vi "Laurel StandAlone TCP.vi"() -> ()   [LabVIEW 2020]
uses:
  Type Definitions/Laurel Serial Commands.ctl
  Type Definitions/Laurel Display Type.ctl
  Type Definitions/Laurel Connection Type.ctl
panel:
  out "appended array":errorcluster[](array[cluster])
  in  "Display Type":T1
  out "Loop Counter":i32
  in  "stop":bool
  out "Single Item":dbl
  out "Gallons (Item 2)":dbl
  out "Flow Rate (Item 1)":dbl format="%.2f"
  in  "All Items Byte Count (Flow Rate)":i32=17
  in  "byte count (Individual)":i32=9
  in  "Laurel Serial Commands":T2
  out "read buffer":string
  out "Error Out 2":errorcluster
  in  "Error In 2":errorcluster
  in  "Hot Laurel Only":string="10.2.0.23"
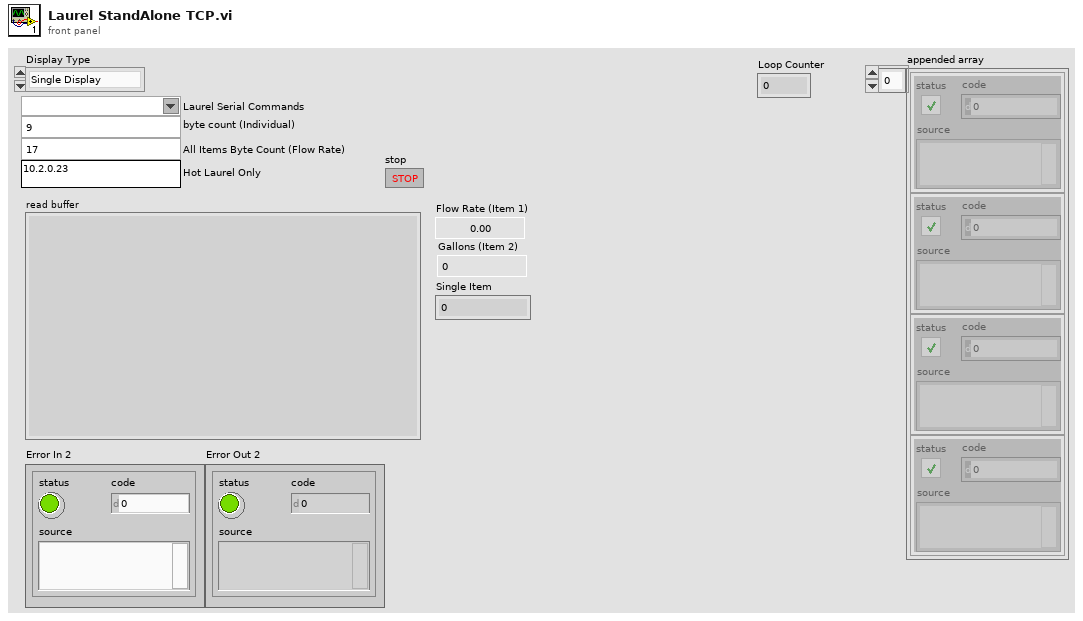
[diagram p1: front panel]
types:
  T1 = typedef "Laurel Display Type.ctl" = enum16{"Single Display", "Dual Display"}
  T2 = typedef "Laurel Serial Commands.ctl" = string
  T3 = typedef "Laurel Connection Type.ctl" = enum16{"Serial", "TCP"}
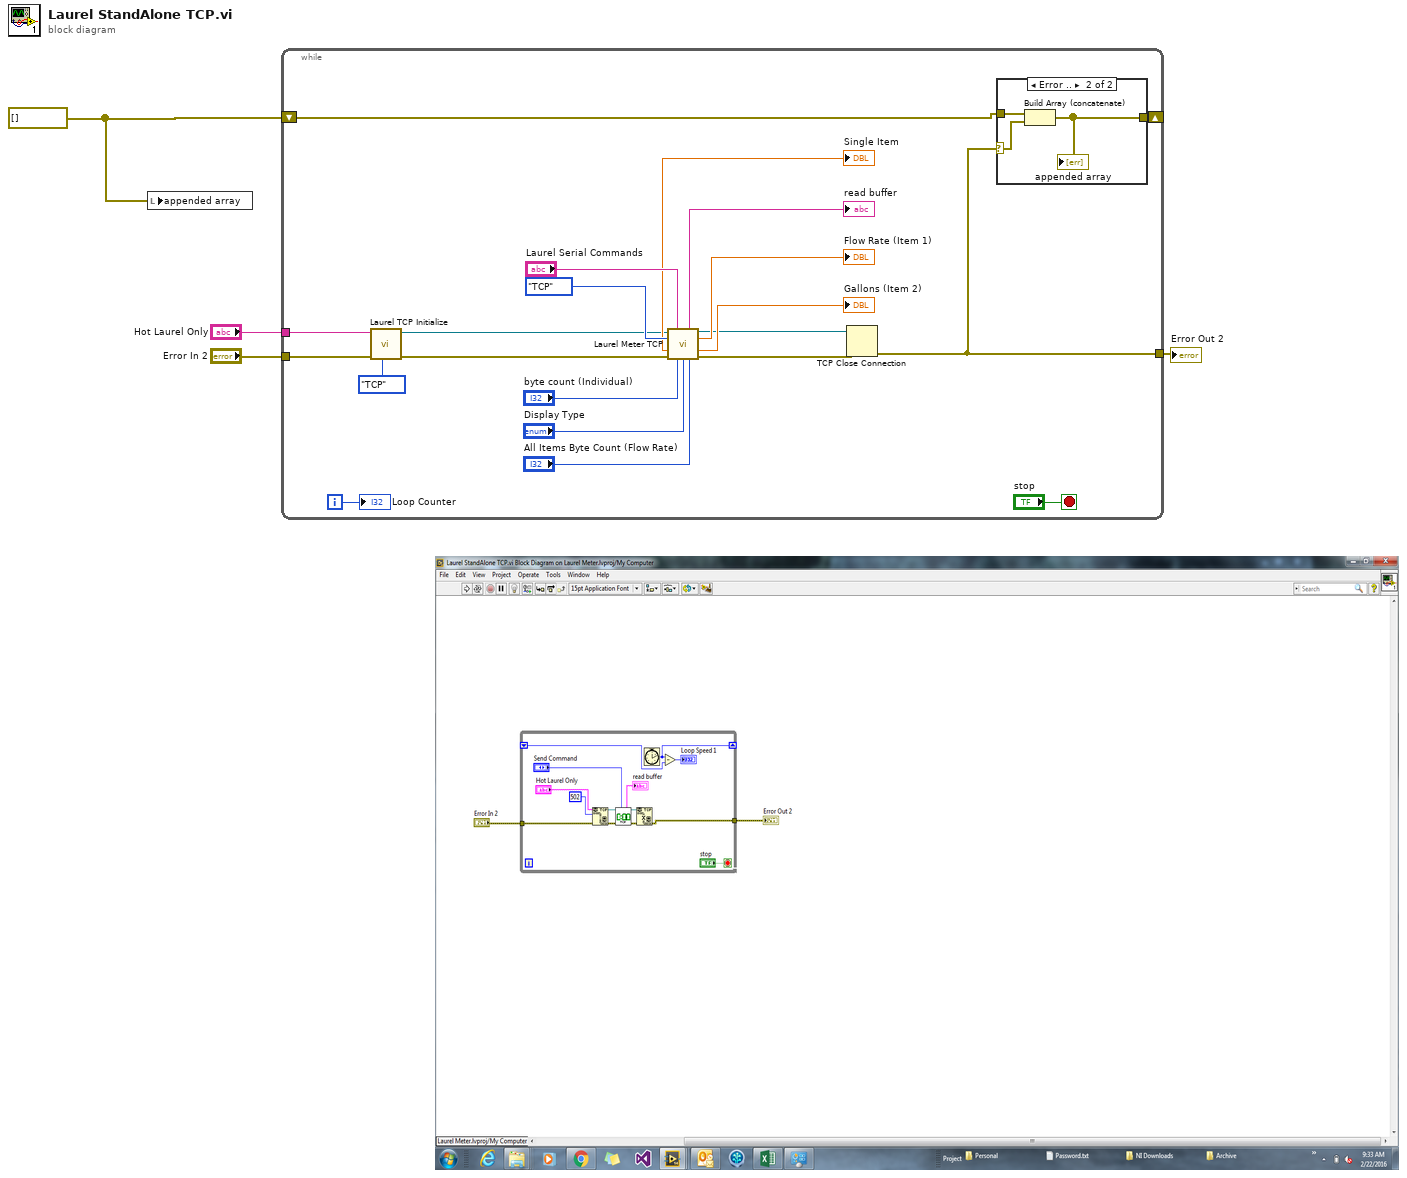
[diagram p0: block diagram]
diagram:
  w1 = errorcluster[] []
  n1 = local write "appended array"(w1) -> ()
  n2 = while {
    tunnel: "Error In 2" -> [w8]
    tunnel: "Hot Laurel Only" -> [w9]
    tunnel: [w11] -> w2
    shift-right: [w10] -> _
    shift-left: w1 -> [w12]
    i -> [w16]
    stop <- "stop" stop-if-true
    n3 = call "Laurel TCP Initialize.vi"("Connection Type"=Laurel_Connection_Type."TCP", "Error In"=w8, "Laurel IP Address"=w9) -> ("Error Out"=w6:errorcluster, "Laurel Ref"=w7:refnum<k5>)  [unwired: 6 in, 1 out]
    n4 = call "Laurel Meter TCP.vi"("TCP Network Connection in"=w7, "Laurel Serial Commands"="Laurel Serial Commands", "Connection Type"=Laurel_Connection_Type."TCP", "error in (no error)"=w6, "byte count (Individual)"="byte count (Individual)", "Display Type"="Display Type", "All Items Byte Count (Flow Rate)"="All Items Byte Count (Flow Rate)") -> ("read buffer"=→"read buffer":string, "TCP Network Connection out"=w13:refnum<k5>, "Flow Rate (Item 1)"=→"Flow Rate (Item 1)":dbl, "Single Item"=→"Single Item":dbl, "Gallons (Item 2)"=→"Gallons (Item 2)":dbl, "error out"=w14:errorcluster)  [unwired: 2 in, 1 out]
    n5 = TCP Close Connection(connection ID=w13, error in (no error)=w14) -> (error out=w11:errorcluster)  [unwired: 1 in, 1 out]
    n6 = case shown="Error .." w11 {
      selector: w11 -> [_ w28]
      tunnel: w12 -> [w26 w29]
      tunnel: [w26 w27] -> w10
      frame No Error {
      }
      frame Error {
        n7 = Build Array (concatenate)(w29, w28) -> (w27:errorcluster[])
        "appended array" <- w27
      }
    }
    "Loop Counter" <- w16
  }
  "Error Out 2" <- w2
